vi "VideoCapture Retrieve.vi"(8 "error in (no error)":errorcluster, 9 "flag":i32, 10 "Image":T1, 11 "VideoCapture in":refnum<class "VideoCapture.lvclass">) -> (0 "error out":errorcluster, 1 "Success":bool, 2 "Image out":T1, 3 "VideoCapture out":refnum<class "VideoCapture.lvclass">)   [LabVIEW 2020, in "OpenLvVision_OpenCv.lvlib" / "VideoCapture.lvclass"]
doc: "Decodes and returns the grabbed video frame."
uses:
  VideoCapture.lvclass
  C:/Users/lukas/Downloads/OpenLvVision_OpenCv/SourceCode/LabView/OpenLvVision_OpenCv/_LvHelpers/EdvrObject/EdvrObject.lvclass
  <vilib>/vision/Image Controls.llb/IMAQ Image.ctl
  _LvHelpers/EdvrObject/EdvrObject.lvclass/EdvrObject.ctl
  OpenLvVision_OpenCv.lvlib
  _LvHelpers/EdvrObject/EdvrObject.lvclass
  Dlls/OlvOpenCvWrapper.dll
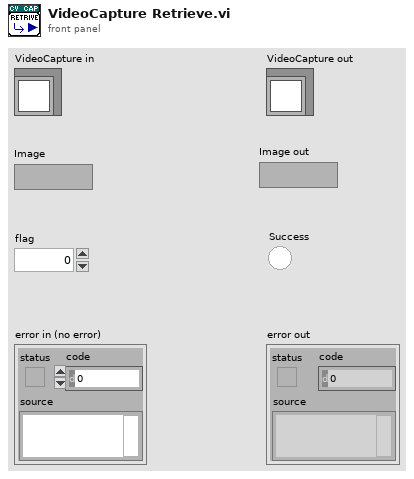
[diagram p1: front panel]
types:
  T1 = typedef "IMAQ Image.ctl" = refnum<image>
  T2 = typedef "OpenLvVision_OpenCv.lvlib/EdvrObject.lvclass/Edvr.ctl" = refnum<data-value>
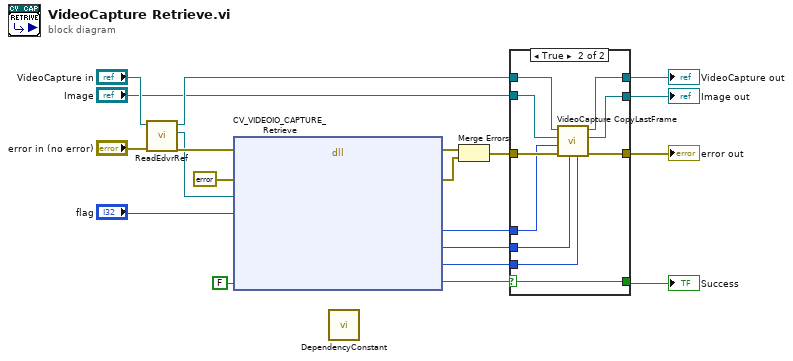
[diagram p0: block diagram]
diagram:
  n1 = call "ReadEdvrRef.vi"("error in (no error)"="error in (no error)", "EdvrObject in"="VideoCapture in") -> ("error out"=w19:errorcluster, "Edvr"=w18:T2, "EdvrObject out"=w13:refnum<class "VideoCapture.lvclass">)  [unwired: 7 in]
  n2 = dll-call lib="C:/Users/lukas/Downloads/OpenLvVision_OpenCv/SourceCode/LabView/OpenLvVision_OpenCv/Dlls/OlvOpenCvWrapper.dll" fn="CV_VIDEOIO_CAPTURE_Retrieve"(error in=w19, "Error"=errorcluster {"status"=FALSE, "code"=0, "source"=""} ("error out"), "edvrRef"=w18, "flags"="flag", "result"=FALSE) -> (error out=w17:errorcluster, "Error"=w16:errorcluster, "width"=w11:i32, "height"=w10:i32, "imageType"=w9:i32, "result"=w14:bool)  [unwired: 8 in, 1 out]
  n3 = call "DependencyConstant.vi"() -> ()  [unwired: 12 in]
  n4 = Merge Errors(w17, w16) -> (w15:errorcluster)
  n5 = case shown="True" w14 {
    selector: w14 -> [w21 w30]
    tunnel: w15 -> [w22 w29]
    tunnel: [w22 w34] -> w6
    tunnel: w13 -> [w24 w33]
    tunnel: [w24 w32] -> w4
    tunnel: [w23 w31] -> w5
    tunnel: "Image" -> [w23 w25]
    tunnel: [w21 w30] -> w7
    tunnel: w11 -> [_ w28]
    tunnel: w10 -> [_ w27]
    tunnel: w9 -> [_ w26]
    frame False {
    }
    frame True {
      n6 = call "VideoCapture CopyLastFrame.vi"("Image Type"=w26, "height"=w27, "error in (no error)"=w29, "width"=w28, "Image"=w25, "VideoCapture in"=w33) -> ("error out"=w34:errorcluster, "Image"=w31:T1, "VideoCapture out"=w32:refnum<class "VideoCapture.lvclass">)  [unwired: 3 in]
    }
  }
  "error out" <- w6
  "VideoCapture out" <- w4
  "Success" <- w7
  "Image out" <- w5
